vi "Run Pre Build Checks.vi"(0 "NSIS Installer":refnum<class "NSIS Installer.lvclass">, 11 "error in (no error)":errorcluster) -> (4 "NSIS Installer":refnum<class "NSIS Installer.lvclass">, 15 "error out":errorcluster)   [LabVIEW 2017, in "CL_G3_VIComponentBuilder.lvlib" / "NSIS Installer.lvclass"]
doc: "1. Verfies that the NSIS build engine is installed."
uses:
  NSIS Installer.lvclass
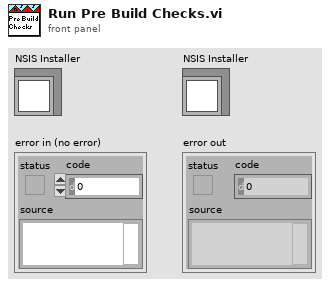
[diagram p1: front panel]
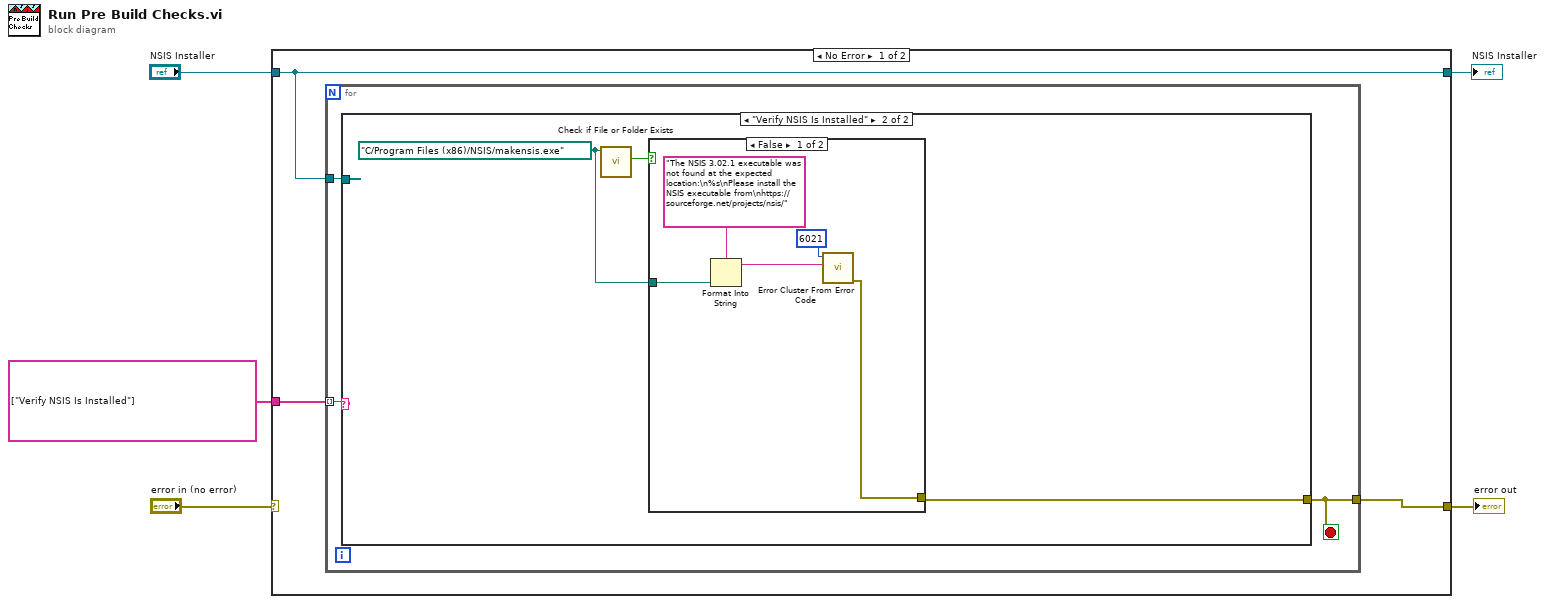
[diagram p0: block diagram]
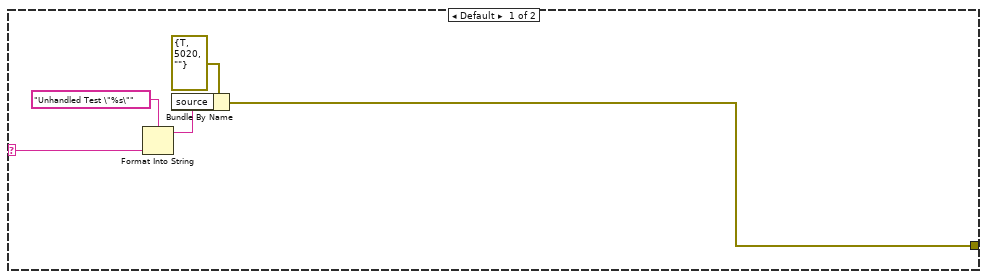
[diagram p2: hidden frame]
diagram:
  n1 = case shown="No Error" "error in (no error)" {
    selector: "error in (no error)" -> [_ w26]
    tunnel: [w7 w26] -> w4
    tunnel: [w8 w25] -> w2
    tunnel: "NSIS Installer" -> [w8 w25]
    tunnel: string[] ["Verify NSIS Is Installed"] -> [w6 _]
    frame No Error {
      n2 = for {
        tunnel: [w11] -> w7
        tunnel: w8 -> [w10]
        tunnel: w6 -> [w9] mode=indexing
        stop <- w11 stop-if-true
        n3 = case shown="\"Verify NSIS Is Installed\"" w9 {
          selector: w9 -> [w13 _]
          tunnel: [w15 w17] -> w11
          tunnel: w10 -> [_ _]
          frame Default {
            n4 = Format Into String(format string="Unhandled Test \"%s\"", w13) -> (resulting string=w12:string)  [unwired: 2 in, 1 out]
            n5 = Bundle By Name(cluster=errorcluster {"status"=TRUE, "code"=5020, "source"=""} ("error out"), "source"=w12) -> (w15:errorcluster)
          }
          frame "Verify NSIS Is Installed" {
            w18 = path "C:/Program Files (x86)/NSIS/makensis.exe" ("path")
            n6 = call <vilib>:"Check if File or Folder Exists.vi"("path"=w18) -> ("file or folder exists?"=w19:bool)  [unwired: 8 in, 2 out]
            n7 = case shown="False" w19 {
              tunnel: w18 -> [w23 _]
              tunnel: [w21 _] -> w17
              frame False {
                n8 = Format Into String(format string="The NSIS 3.02.1 executable was not found at the expected location:\n%s\nPlease install the NSIS executable from\nhttps://sourceforge.net/projects/nsis/", w23) -> (resulting string=w22:string)  [unwired: 2 in, 1 out]
                n9 = call <vilib>:"Error Cluster From Error Code.vi"("error message (\"\")"=w22, "error code (0)"=6021) -> ("error out"=w21:errorcluster)  [unwired: 7 in]
              }
              frame True {
              }
            }
          }
        }
      }
    }
    frame Error {
    }
  }
  "error out" <- w4
  "NSIS Installer" <- w2
